vi "Save_RawImageCSV.vi"(1 "error in (no error)":errorcluster, 2 "Capture number":i32, 3 "Image":dbl[][][](array[numeric]), 4 "TDMS file":refnum<k34>) -> (0 "error in (no error) 2":errorcluster)   [LabVIEW 2018]
uses:
  <vilib>/Utility/file.llb/Write Delimited Spreadsheet (DBL).vi
  <vilib>/Utility/file.llb/Write Delimited Spreadsheet (string).vi
  <vilib>/regexp/Match Regular Expression.xnode
panel:
  out "before match":string
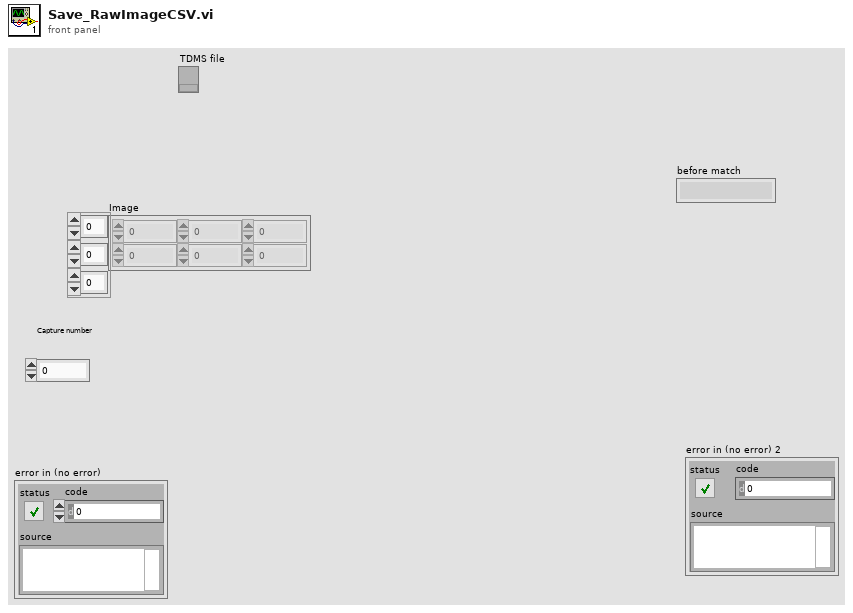
[diagram p1: front panel]
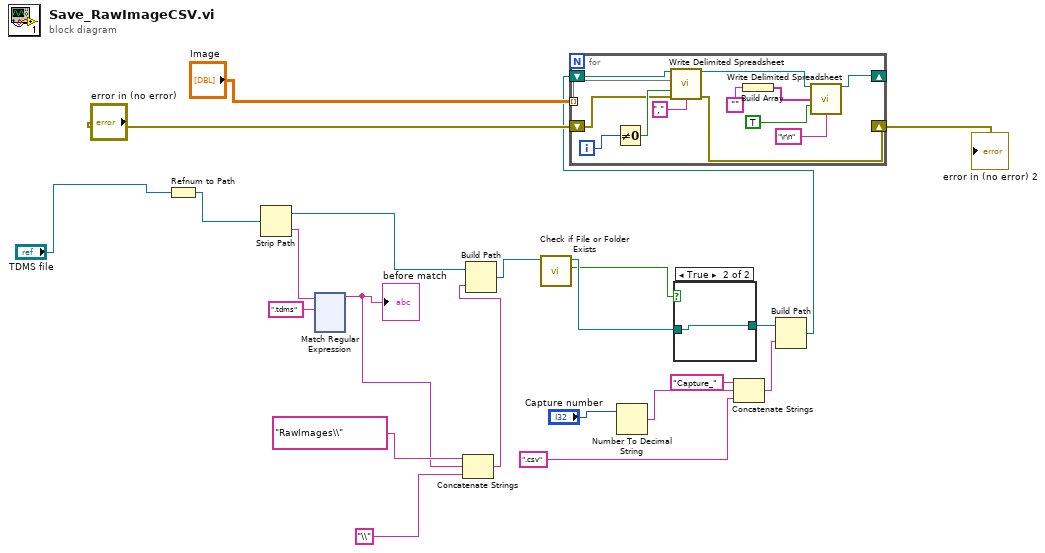
[diagram p0: block diagram]
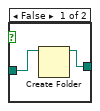
[diagram p2: hidden frame]
diagram:
  n1 = Refnum to Path(1:"TDMS file") -> (0:w20:path)
  n2 = Strip Path(path=w20) -> (stripped path=w19:path, name=w15:string)
  n3 = xnode "Match Regular Expression"("input string"=w15, "regular expression"=".tdms") -> ("before match"=w4:string)  [unwired: 4 in, 4 out]
  "before match" <- w4
  n4 = Concatenate Strings("RawImages\\", w4, "\\" ("string")) -> (w13:string)
  n5 = Build Path(base path=w19, name or relative path=w13) -> (appended path=w9:path)
  n6 = call <vilib>:"Check if File or Folder Exists.vi"("path"=w9) -> ("file or folder exists?"=w7:bool, "dup path"=w8:path)  [unwired: 8 in, 1 out]
  n7 = Number To Decimal String(number="Capture number") -> (decimal integer string=w2:string)  [unwired: 1 in]
  n8 = case shown="True" w7 {
    tunnel: [w24 w25] -> w12
    tunnel: w8 -> [w23 w25]
    frame False {
      n9 = Create Folder(path (use dialog)=w23) -> (created path=w24:path)  [unwired: 2 in, 2 out]
    }
    frame True {
    }
  }
  n10 = Concatenate Strings("Capture_" ("string"), w2, ".csv" ("string")) -> (w11:string)
  n11 = Build Path(base path=w12, name or relative path=w11) -> (appended path=w10:path)
  n12 = for {
    tunnel: "Image" -> [w37] mode=indexing
    shift-right: [w30] -> _
    shift-left: w10 -> [w36]
    shift-right: [w26] -> w6
    shift-left: "error in (no error)" -> [w27]
    i -> [w35]
    n13 = Not Equal To 0?(x=w35) -> (x != 0?=w34:bool)
    n14 = call-poly <vilib>:"Write Delimited Spreadsheet.vi"("file path (dialog if empty)"=w36, "2D data"=w37, "append to file? (new file:F)"=w34, "error in (no error)"=w27, "delimiter (\\t)"="," ("delimiter (\\t)")) -> ("new file path (Not A Path if cancelled)"=w33:path, "error out"=w26:errorcluster)  [unwired: 9 in]
    n15 = Build Array("") -> (w28:string[])
    n16 = call-poly <vilib>:"Write Delimited Spreadsheet.vi"("file path (dialog if empty)"=w33, "1D data"=w28, "append to file? (new file:F)"=TRUE, "delimiter (\\t)"="\r\n" ("delimiter (\\t)")) -> ("new file path (Not A Path if cancelled)"=w30:path)  [unwired: 10 in, 1 out]
  }
  "error in (no error) 2" <- w6
